vi "StringTimeCalculate.vi"(9 "End Date":string="2014/9/21 上午 12:00:01", 11 "Start Date":string="2014/9/20 上午 12:00:00") -> (2 "Minutes":i32, 4 "SQLEndTime":string, 5 "SQLStartTime":string)   [LabVIEW 2012]
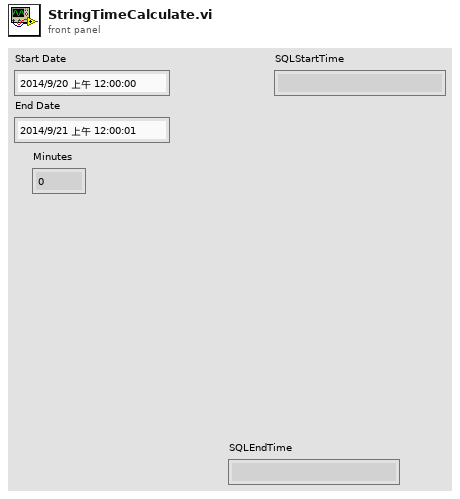
[diagram p1: front panel]
types:
  T1 = typedef "LVDateTimeRec.ctl" = cluster{"fractional second":dbl, "second":i32, "minute":i32, "hour":i32, "day of month":i32, "month":i32, "year":i32, "day of week":i32, "day of year":i32, "DST":i32}
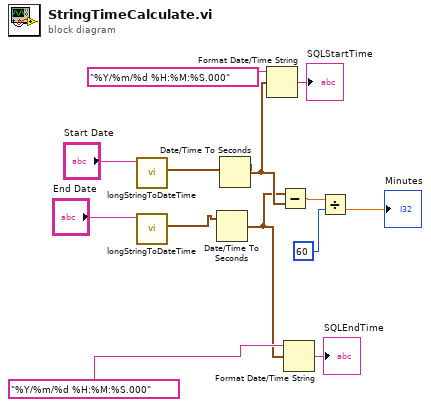
[diagram p0: block diagram]
diagram:
  n1 = call "longStringToDateTime.vi"("input string"="Start Date") -> ("output cluster"=w7:T1)  [unwired: 10 in]
  n2 = call "longStringToDateTime.vi"("input string"="End Date") -> ("output cluster"=w11:T1)  [unwired: 10 in]
  n3 = Date/Time To Seconds(2:w11) -> (0:w1:timestamp)  [unwired: 1 in]
  n4 = Date/Time To Seconds(2:w7) -> (0:w6:timestamp)  [unwired: 1 in]
  n5 = Format Date/Time String(time format string (%c)="%Y/%m/%d %H:%M:%S.000", seconds (now)=w6) -> (date/time string=→"SQLStartTime":string)  [unwired: 1 in]
  n6 = Subtract(x=w1, y=w6) -> (x-y=w8:dbl)
  n7 = Format Date/Time String(time format string (%c)="%Y/%m/%d %H:%M:%S.000", seconds (now)=w1) -> (date/time string=→"SQLEndTime":string)  [unwired: 1 in]
  n8 = Divide(x=w8, y=60) -> (x/y=→"Minutes":dbl)
